vi "Get Image from Clipboard.vi"(6 "error in":errorcluster, 7 "image depth (24)":i32(ring)=24 items=["1"=1, "4"=4, "8"=8, "24"=24]) -> (2 "error out":errorcluster, 3 "image data":T1)   [LabVIEW 2025, in "XNode Support.lvlib"]
uses:
  XNode Support.lvlib
  <vilib>/picture/picture.llb/imagedata.ctl
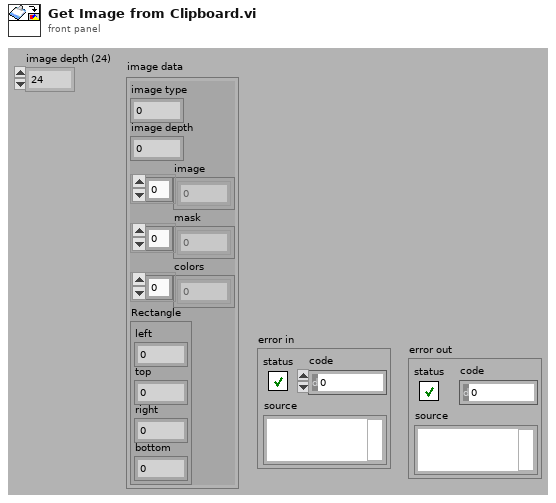
[diagram p1: front panel]
types:
  T1 = typedef "imagedata.ctl" = cluster{"image type":i32, "image depth":i32, "image":u8[], "mask":u8[], "colors":u32[], "Rectangle":cluster{"left":i16, "top":i16, "right":i16, "bottom":i16}}
  T2 = typedef "LVRectTypeDef.ctl" = cluster{"Left":i16, "Top":i16, "Right":i16, "Bottom":i16}
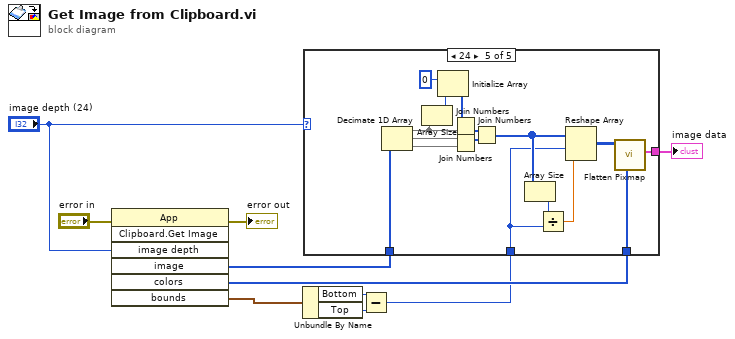
[diagram p0: block diagram]
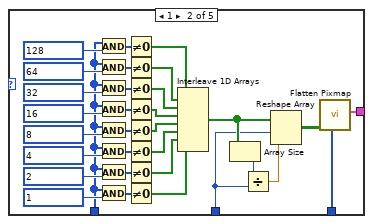
[diagram p3: hidden frame]
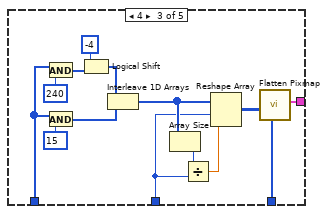
[diagram p4: hidden frame]
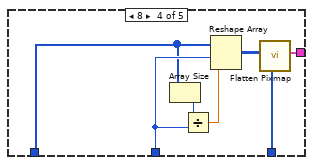
[diagram p5: hidden frame]
diagram:
  n1 = invoke class="App" method="Clipboard.Get Image"(error in="error in", "image depth"="image depth (24)") -> (error out=→"error out":errorcluster, "image"=w3:u8[], "colors"=w6:u32[], "bounds"=w10:T2)  [unwired: 5 in, 3 out]
  n2 = Unbundle By Name(w10) -> ("Bottom"=w9:i16, "Top"=w8:i16)
  n3 = Subtract(x=w9, y=w8) -> (x-y=w5:i16)
  n4 = case shown="24" "image depth (24)" {
    tunnel: [_ w14 w44 w60 w79] -> w7
    tunnel: w6 -> [_ w11 w43 w59 w69]
    tunnel: w3 -> [_ w13 w46 w57 w65]
    tunnel: w5 -> [_ w12 w45 w58 w64]
    frame Default {
    }
    frame 1 {
      n5 = And(x=w13, y=u8 128) -> (x .and. y?=w26:u8[])
      n6 = And(x=w13, y=u8 64) -> (x .and. y?=w27:u8[])
      n7 = And(x=w13, y=u8 32) -> (x .and. y?=w28:u8[])
      n8 = And(x=w13, y=u8 16) -> (x .and. y?=w29:u8[])
      n9 = And(x=w13, y=8) -> (x .and. y?=w30:i32[])
      n10 = And(x=w13, y=u8 4) -> (x .and. y?=w31:u8[])
      n11 = And(x=w13, y=u8 2) -> (x .and. y?=w32:u8[])
      n12 = And(x=w13, y=u8 1) -> (x .and. y?=w33:u8[])
      n13 = Not Equal To 0?(x=w26) -> (x != 0?=w34:bool[])
      n14 = Not Equal To 0?(x=w27) -> (x != 0?=w36:bool[])
      n15 = Not Equal To 0?(x=w28) -> (x != 0?=w38:bool[])
      n16 = Not Equal To 0?(x=w29) -> (x != 0?=w41:bool[])
      n17 = Not Equal To 0?(x=w30) -> (x != 0?=w40:bool[])
      n18 = Not Equal To 0?(x=w31) -> (x != 0?=w39:bool[])
      n19 = Not Equal To 0?(x=w32) -> (x != 0?=w37:bool[])
      n20 = Not Equal To 0?(x=w33) -> (x != 0?=w35:bool[])
      n21 = Interleave 1D Arrays(w34, w36, w38, w41, w40, w39, w37, w35) -> (w42:bool[])
      n22 = Array Size(array=w42) -> (size(s)=w15:i32)
      n23 = Divide(x=w15, y=w12) -> (x/y=w16:dbl)
      n24 = Reshape Array(w42, w12, w16) -> (w17:bool[][])
      n25 = call <vilib>:"Flatten Pixmap.vi"("colors"=w11, "1-bit pixmap"=w17) -> ("image data"=w14:T1)  [unwired: 9 in]
    }
    frame 4 {
      n26 = And(x=w46, y=u8 240) -> (x .and. y?=w49:u8[])
      n27 = And(x=w46, y=u8 15) -> (x .and. y?=w52:u8[])
      n28 = Logical Shift(y=-4, x=w49) -> (x << y=w51:u8[])
      n29 = Interleave 1D Arrays(w51, w52) -> (w55:u8[])
      n30 = Array Size(array=w55) -> (size(s)=w54:i32)
      n31 = Divide(x=w54, y=w45) -> (x/y=w56:dbl)
      n32 = Reshape Array(w55, w45, w56) -> (w53:u8[][])
      n33 = call <vilib>:"Flatten Pixmap.vi"("colors"=w43, "4-bit pixmap"=w53) -> ("image data"=w44:T1)  [unwired: 9 in]
    }
    frame 8 {
      n34 = Array Size(array=w57) -> (size(s)=w62:i32)
      n35 = Divide(x=w62, y=w58) -> (x/y=w63:dbl)
      n36 = Reshape Array(w57, w58, w63) -> (w61:u8[][])
      n37 = call <vilib>:"Flatten Pixmap.vi"("colors"=w59, "8-bit pixmap"=w61) -> ("image data"=w60:T1)  [unwired: 9 in]
    }
    frame 24 {
      n38 = Decimate 1D Array(w65) -> (w71:u8[], w78:u8[], w77:u8[])
      n39 = Array Size(array=w71) -> (size(s)=w72:i32)
      n40 = Initialize Array(u8 0, w72) -> (w70:u8[])
      n41 = Join Numbers(hi=w70, lo=w71) -> ((hi.lo)=w76:u16[])
      n42 = Join Numbers(hi=w78, lo=w77) -> ((hi.lo)=w75:u16[])
      n43 = Join Numbers(hi=w76, lo=w75) -> ((hi.lo)=w67:u32[])
      n44 = Array Size(array=w67) -> (size(s)=w68:i32)
      n45 = Divide(x=w68, y=w64) -> (x/y=w66:dbl)
      n46 = Reshape Array(w67, w64, w66) -> (w74:u32[][])
      n47 = call <vilib>:"Flatten Pixmap.vi"("colors"=w69, "24-bit pixmap"=w74) -> ("image data"=w79:T1)  [unwired: 9 in]
    }
  }
  "image data" <- w7
